vi "BuildRequestFilter.vi"(6 "InputCondition":string, 7 "Filter":T1, 8 "error in":errorcluster, 9 "Filter Text":string, 10 "To":timestamp, 11 "From":timestamp) -> (0 "error out":errorcluster, 2 "condition":string)   [LabVIEW 2015, in "DatabaseApi.lvlib"]
uses:
  DatabaseApi.lvlib
  TypeDef/RequestsTableColumnNamesRing.ctl
  TypeDef/RequestsTableDbTableName.ctl
  <vilib>/addons/database/Connection.llb/DB Tools Open Connec (Path).vi
  <vilib>/addons/database/Auxilliary.llb/DB Tools Format Datetime String (Time Stamp).vi
  <vilib>/regexp/Match Regular Expression.xnode
  <vilib>/addons/database/NI_Database_API.lvlib
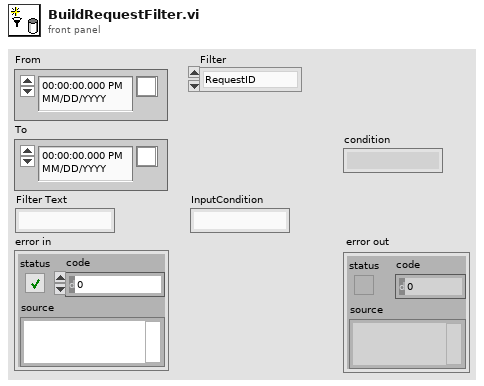
[diagram p1: front panel]
types:
  T1 = typedef "DatabaseApi.lvlib/RequestsTableColumnNamesRing.ctl" = enum16{"RequestID", "PersonnelType", "StartTime", "StartName", "AckTime", "AckName", "FulfilledTime", "FulfilledName", "Description"}
  T2 = typedef "DatabaseApi.lvlib/RequestsTableDbTableName.ctl" = string
  T3 = typedef "NI_Database_API.lvlib/Conn ObjectReference.ctl" = refnum<k1>
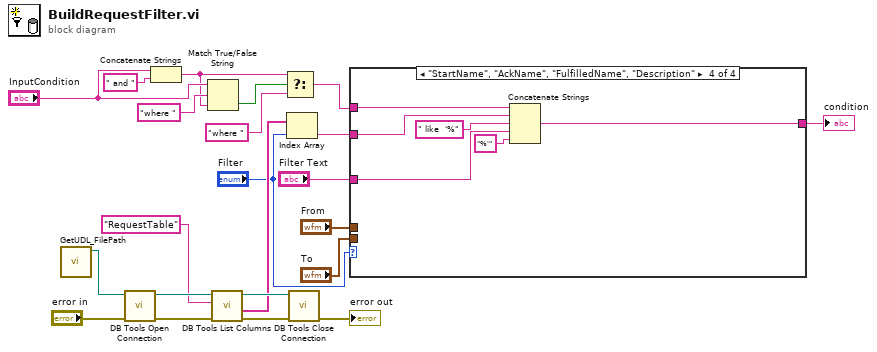
[diagram p0: block diagram]
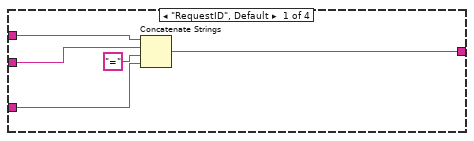
[diagram p2: hidden frame]
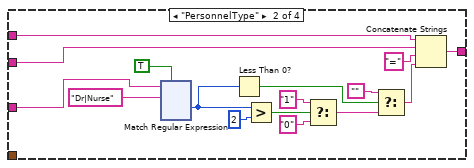
[diagram p3: hidden frame]
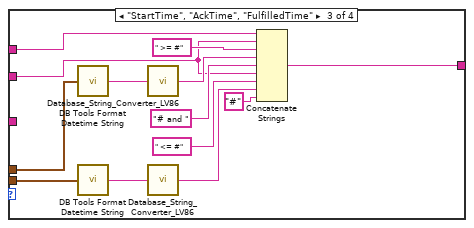
[diagram p4: hidden frame]
diagram:
  n1 = call "GetUDL_FilePath.vi"() -> ("UDL file path"=w20:path)  [unwired: 11 in]
  n2 = call-poly <vilib>:"DB Tools Open Connection.vi"("error in (no error)"="error in", "connection information"=w20) -> ("error out"=w19:errorcluster, "connection reference"=w17:T3)  [unwired: 6 in]
  n3 = Concatenate Strings("InputCondition", " and " ("string")) -> (w2:string)
  n4 = Match True/False String(2:w2, 3:"where " ("string"), 4:"InputCondition") -> (0:w5:bool)  [unwired: 1 out]
  n5 = call <vilib>:"DB Tools List Columns.vi"("error in (no error)"=w19, "table"=T2 "RequestTable", "connection reference"=w17) -> ("error out"=w15:errorcluster, "columns"=w12:string[], "connection reference out"=w14:T3)  [unwired: 1 in, 1 out]
  n6 = Select(t=w2, s=w5, f="where " ("string")) -> (s? t:f=w4:string)
  n7 = Index Array(array=w12, index="Filter") -> (element=w8:string)
  n8 = call <vilib>:"DB Tools Close Connection.vi"("error in (no error)"=w15, "connection reference"=w14) -> ("error out"=→"error out":errorcluster)  [unwired: 5 in]
  n9 = case shown="\"StartName\", \"AckName\", \"FulfilledName\", \"Description\"" "Filter" {
    tunnel: "To" -> [_ _ w170 _]
    tunnel: "From" -> [_ _ w169 _]
    tunnel: [w24 w41 w166 w175] -> w10
    tunnel: "Filter Text" -> [w26 w39 _ w174]
    tunnel: w8 -> [w27 w42 w162 w172]
    tunnel: w4 -> [w23 w28 w158 w171]
    frame "RequestID", Default {
      n10 = Concatenate Strings(w23, w27, "=" ("string"), w26) -> (w24:string)
    }
    frame "PersonnelType" {
      n11 = xnode "Match Regular Expression"("input string"=w39, "regular expression"="Dr|Nurse", "ignore case? (F)"=TRUE) -> ("offset past match"=w34:i32)  [unwired: 3 in, 4 out]
      n12 = Less Than 0?(x=w34) -> (x < 0?=w37:bool)
      n13 = Greater?(x=w34, y=2) -> (0:w32:bool)
      n14 = Select(t="1" ("string"), s=w32, f="0" ("string")) -> (s? t:f=w30:string)
      n15 = Select(t="" ("string"), s=w37, f=w30) -> (s? t:f=w35:string)
      n16 = Concatenate Strings(w28, w42, "=" ("string"), w35) -> (w41:string)
    }
    frame "StartTime", "AckTime", "FulfilledTime" {
      n17 = call-poly <vilib>:"DB Tools Format Datetime String.vi"("time stamp"=w169) -> ("date/time string"=w168:string)
      n18 = call-poly <vilib>:"DB Tools Format Datetime String.vi"("time stamp"=w170) -> ("date/time string"=w164:string)
      n19 = call "Database_String_Converter_LV86.vi"("String Input (date/timeyyyy-mm-dd hh:mm:ss)"=w168) -> ("String Output (mm/dd/yyyy hh:mm:ss AM/PM)"=w163:string)  [unwired: 4 in]
      n20 = call "Database_String_Converter_LV86.vi"("String Input (date/timeyyyy-mm-dd hh:mm:ss)"=w164) -> ("String Output (mm/dd/yyyy hh:mm:ss AM/PM)"=w161:string)  [unwired: 4 in]
      n21 = Concatenate Strings(w158, w162, " >= #" ("string"), w163, "# and " ("string"), w162, " <= #" ("string"), w161, "#" ("string")) -> (w166:string)
    }
    frame "StartName", "AckName", "FulfilledName", "Description" {
      n22 = Concatenate Strings(w171, w172, " like  '%" ("string"), w174, "%'" ("string")) -> (w175:string)
    }
  }
  "condition" <- w10
